vi "Format Test Result Query.vi"(8 "error in (no error)":errorcluster, 9 "Serial Number":string, 10 "Part Number":string, 11 "NI Skyline Configuration HTTP in":refnum<class "NI Skyline Configuration HTTP.lvclass">) -> (0 "error out":errorcluster, 1 "String":string, 2 "String 2":string, 3 "http session":T1)   [LabVIEW 2019]
uses:
  <vilib>/Skyline/Configuration/Configuration HTTP_class/NI Skyline Configuration HTTP.lvclass
  <vilib>/httpClient/ClientHandle.ctl
  <vilib>/Skyline/Configuration/Configuration HTTP_class/NI Skyline Configuration HTTP.lvclass/NI Skyline Configuration HTTP.ctl
  <vilib>/Skyline/Configuration/Configuration HTTP_class/Read Server URL.vi
  <vilib>/httpClient/LabVIEWHTTPClient.lvlib
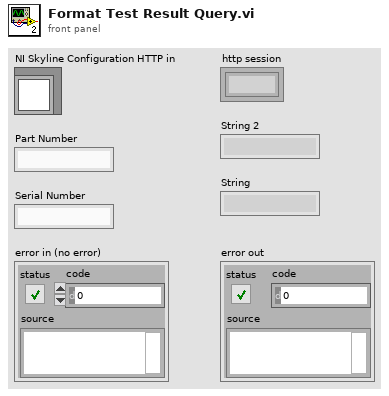
[diagram p1: front panel]
types:
  T1 = typedef "LabVIEWHTTPClient.lvlib/ClientHandle.ctl" = refnum<k1>
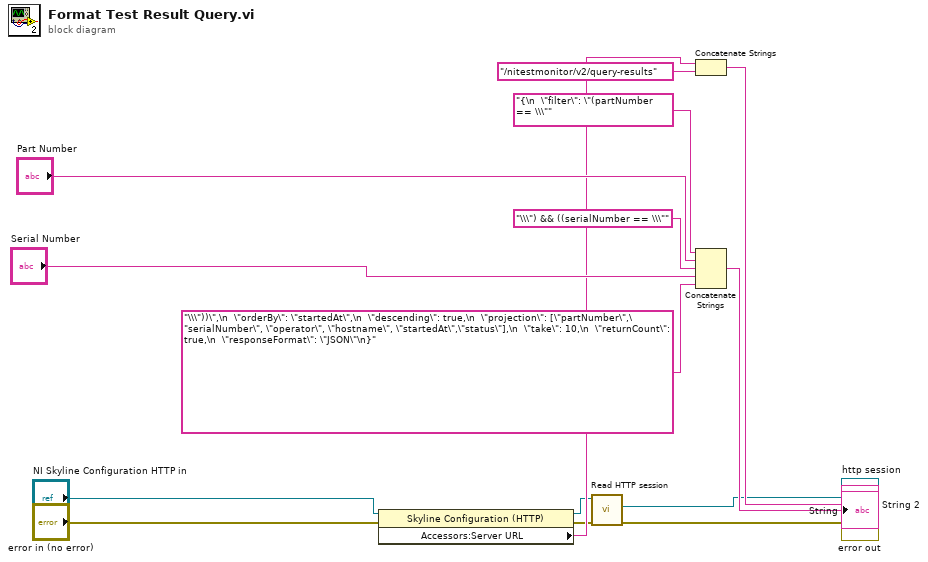
[diagram p0: block diagram]
diagram:
  n1 = property class="Skyline Configuration (HTTP)"(reference="NI Skyline Configuration HTTP in", error in="error in (no error)") -> (reference out=w4:refnum<class "NI Skyline Configuration HTTP.lvclass">, error out=w5:errorcluster, "Accessors:Server URL"=w7:string)
  n2 = call <vilib>:"Read HTTP session.vi"("error in (no error)"=w5, "HTTP configuration in"=w4) -> ("error out"=→"error out":errorcluster, "http session"=→"http session":T1)  [unwired: 7 in, 1 out]
  n3 = Concatenate Strings(w7, "/nitestmonitor/v2/query-results" ("string")) -> (→"String 2":string)
  n4 = Concatenate Strings("{\n  \"filter\": \"(partNumber == \\\"" ("buffer"), "Part Number", "\\\") && ((serialNumber == \\\"" ("buffer"), "Serial Number", "\\\"))\",\n  \"orderBy\": \"startedAt\",\n  \"descending\": true,\n  \"projection\": [\"partNumber\",\"serialNumber\", \"operator\", \"hostname\", \"startedAt\",\"status\"],\n  \"take\": 10,\n  \"returnCount\": true,\n  \"responseFormat\": \"JSON\"\n}" ("string")) -> (→"String":string)
